vi "Construct Advanced Text Log Sink.vi"(7 "LogLevel":T3, 8 "StringFormat":refnum<class "IStringFormat.lvclass">, 9 "Log Filter":refnum<class "ILogFilter.lvclass">, 10 "Error Action":T1=enum."Ignore Error and Close Sink", 11 "Text File Configuration":T2={"Folder"=path "", "Name"="Event Log", "Extension"="txt", "Max Size (MB)"=1, "Timestamp Filename"=TRUE}) -> (3 "Text File Sink out":refnum<class "Text File Sink.lvclass">)   [LabVIEW 2020, in "Text File Sink.lvclass"]
doc: "Construct a text file sink. Text file configuration parameters are defined below.\n-Folder - the folder path where log files will be generated. If an empty path is supplied, a default folder path at public application data will be used.\n-Name - Name to give the log file. If no name is provided, a default file name cooresponding to the application directory name will be used.\n-Extension - file extension to be used for the log file. Note a period is not required here."
uses:
  <vilib>/gpm_packages/@cs/event-logger/Source/Text File Sink/Text File Sink.lvclass
  C:/Program Files/National Instruments/LabVIEW 2020/vi.lib/gpm_packages/@cs/event-logger/Source/Composed Log/Log Sink/Log Sink.lvclass
  C:/Program Files/National Instruments/LabVIEW 2020/vi.lib/gpm_packages/@cs/event-logger/Source/String Log Sink/String Log Sink.lvclass
  <vilib>/gpm_packages/@cs/event-logger/Source/Composed Log/Types/Log Level.ctl
  <vilib>/gpm_packages/@cs/event-logger/Source/Text File Sink/Configuration.ctl
  <vilib>/gpm_packages/@cs/event-logger/Source/Composed Log/Log Sink/Sink Error Actions ENUM.ctl
  <vilib>/gpm_packages/@cs/event-logger/Source/Composed Log/ILogFilter/ILogFilter.lvclass
  <vilib>/gpm_packages/@cs/event-logger/Source/IStringFormat/IStringFormat.lvclass
  <vilib>/Utility/sysdir.llb/System Directory Type.ctl
  <vilib>/gpm_packages/@cs/event-logger/Source/Text File Sink/Text File Sink.lvclass/Text File Sink.ctl
  <vilib>/gpm_packages/@cs/event-logger/Source/Composed Log/Log Sink/Log Sink.lvclass/Log Sink.ctl
  <vilib>/gpm_packages/@cs/event-logger/Source/String Log Sink/String Log Sink.lvclass/String Log Sink.ctl
  <vilib>/gpm_packages/@cs/event-logger/Source/Composed Log/Log Sink/Log Sink.lvclass
  <vilib>/gpm_packages/@cs/event-logger/Source/String Log Sink/String Log Sink.lvclass
  <vilib>/gpm_packages/@cs/event-logger/Source/Composed Log/Composed Log.lvlib
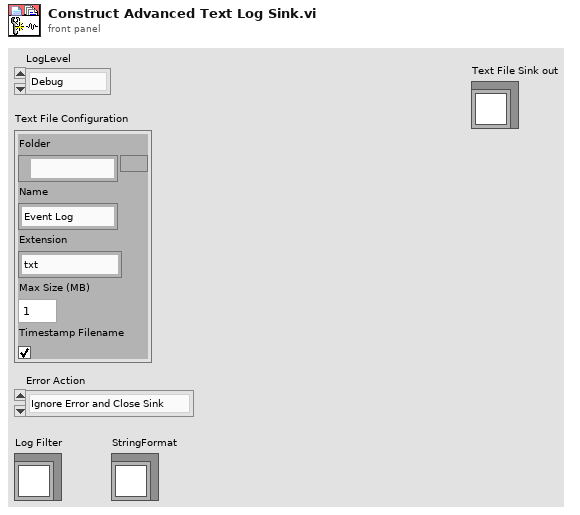
[diagram p1: front panel]
types:
  T1 = typedef "Composed Log.lvlib/Log Sink.lvclass/Sink Error Actions ENUM.ctl" = enum16{"Ignore Error and Continue", "Ignore Error and Close Sink", "Report Error and Close Sink"}
  T2 = typedef "Text File Sink.lvclass/Configuration.ctl" = cluster{"Folder":path, "Name":string, "Extension":string, "Max Size (MB)":i64, "Timestamp Filename":bool}
  T3 = typedef "Composed Log.lvlib/Log Level.ctl" = enum16{"Debug", "Info", "Warning", "Error", "Critical"}
  T4 = typedef "System Directory Type.ctl" = i32
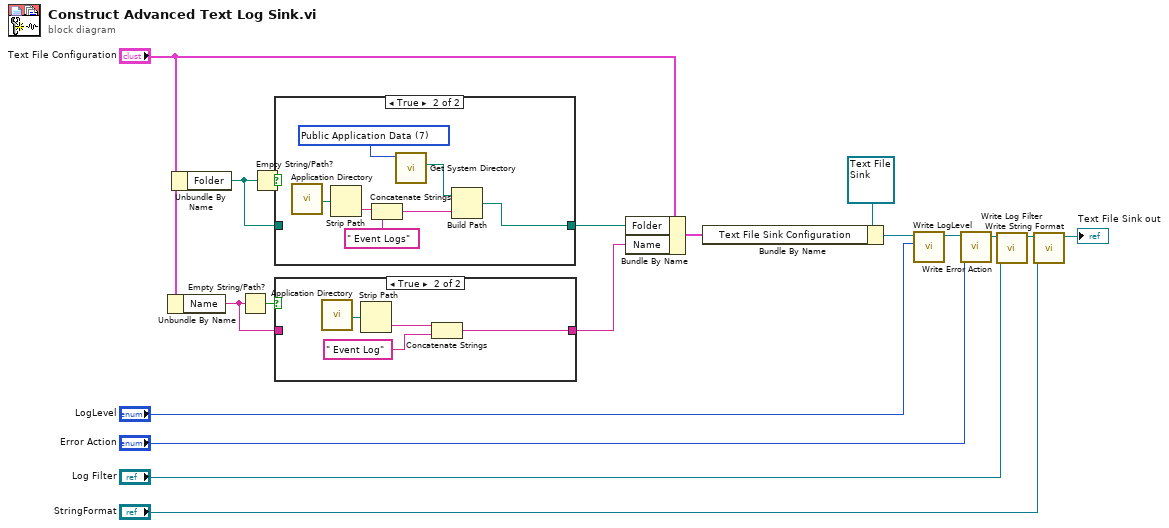
[diagram p0: block diagram]
diagram:
  n1 = Unbundle By Name("Text File Configuration") -> ("Name"=w9:string)
  n2 = Unbundle By Name("Text File Configuration") -> ("Folder"=w11:path)
  n3 = Empty String/Path?(string/path=w9) -> (empty?=w14:bool)
  n4 = Empty String/Path?(string/path=w11) -> (empty?=w16:bool)
  n5 = case shown="True" w16 {
    tunnel: w11 -> [w19 _]
    tunnel: [w19 w20] -> w15
    frame False {
    }
    frame True {
      w26 = T4 7 items=["User Home"=0, "User Desktop"=1, "User Documents"=2, "User Application Data"=3, "User Preferences"=4, "User Temporary"=5, "Public Documents"=6, "Public Application Data"=7, "Public Preferences"=8, "Public Cache"=13, "System Core Libraries"=9, "System Installed Libraries"=10, "Application Files"=11, "Boot Volume Root"=12] ("system directory type")
      n6 = call <vilib>:"Application Directory.vi"() -> ("Application Directory"=w25:path)
      n7 = Strip Path(path=w25) -> (name=w24:string)  [unwired: 1 out]
      n8 = Concatenate Strings(w24, " Event Logs" ("string")) -> (w22:string)
      n9 = call <vilib>:"Get System Directory.vi"("system directory type"=w26) -> ("system directory"=w21:path)  [unwired: 10 in]
      n10 = Build Path(base path=w21, name or relative path=w22) -> (appended path=w20:path)
    }
  }
  n11 = case shown="True" w14 {
    tunnel: w9 -> [w27 _]
    tunnel: [w27 w28] -> w13
    frame False {
    }
    frame True {
      n12 = call <vilib>:"Application Directory.vi"() -> ("Application Directory"=w31:path)
      n13 = Strip Path(path=w31) -> (name=w30:string)  [unwired: 1 out]
      n14 = Concatenate Strings(w30, " Event Log" ("string")) -> (w28:string)
    }
  }
  n15 = Bundle By Name(cluster="Text File Configuration", "Folder"=w15, "Name"=w13) -> (w8:T2)
  n16 = Bundle By Name(cluster=refnum<class "Text File Sink.lvclass"> refnum ("Text File Sink in"), "Text File Sink Configuration"=w8) -> (w12:refnum<class "Text File Sink.lvclass">)
  n17 = call <vilib>:"Write LogLevel.vi"("LogLevel"="LogLevel", "Log Sink in"=w12) -> ("Log Sink out"=w6:refnum<class "Text File Sink.lvclass">)  [unwired: 8 in, 1 out]
  n18 = call <vilib>:"Write Error Action.vi"("Error Action"="Error Action", "Log Sink in"=w6) -> ("Log Sink out"=w7:refnum<class "Text File Sink.lvclass">)  [unwired: 8 in, 1 out]
  n19 = call <vilib>:"Write Log Filter.vi"("Log Filter"="Log Filter", "Log Sink in"=w7) -> ("Log Sink out"=w3:refnum<class "Text File Sink.lvclass">)  [unwired: 8 in, 1 out]
  n20 = call <vilib>:"Write String Format.vi"("StringFormat"="StringFormat", "String Log Sink in"=w3) -> ("String Log Sink out"=→"Text File Sink out":refnum<class "Text File Sink.lvclass">)  [unwired: 8 in, 1 out]
